vi "getSheetDim.vi"(8 "error in (no error)":errorcluster, 10 "Refnum Cluster Out":T1, 11 "reference in":refnum<class "excelFile.lvclass">) -> (0 "error out":errorcluster, 2 "rowNumber":i32, 3 "reference out":refnum<class "excelFile.lvclass">)   [LabVIEW 2015, in "excelFile.lvclass"]
uses:
  excelFile.lvclass
  <userlib>/Read_Excel_Values.llb/GetXL_CellValues_2D_String.vi
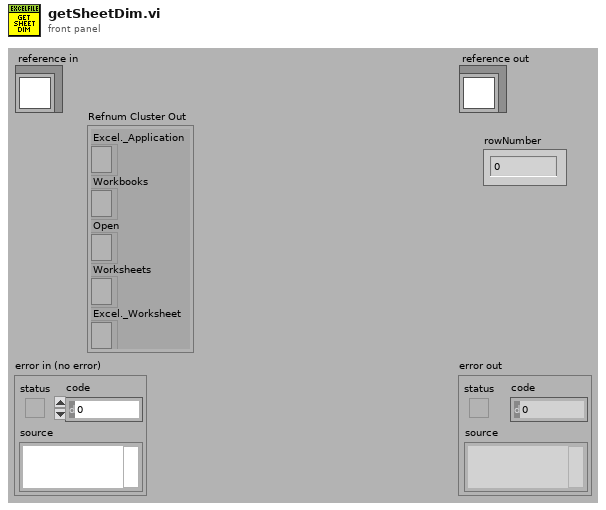
[diagram p1: front panel]
types:
  T1 = cluster{"Excel._Application":refnum<k7>, "Workbooks":refnum<k7>, "Open":refnum<k7>, "Worksheets":refnum<k7>, "Excel._Worksheet":refnum<k7>}
  T2 = typedef "excelFile.lvclass/ObjectAttributesRef.ctl" = refnum<data-value>
  T3 = typedef "excelFile.lvclass/ObjectAttributes.ctl" = cluster{"MyAttribute":dbl, "path":string, "Refnum Excel":cluster{"Excel._Application":refnum<k7>, "Workbooks":refnum<k7>, "Open":refnum<k7>}, "data":string[][][], "fileType":T4, "sheetName":string[]}
  T4 = typedef "excelFile.lvclass/fileType.ctl" = enum16{"database", "CosmedTest"}
  T5 = cluster{"Excel._Application":refnum<k7>, "Workbooks":refnum<k7>, "Open":refnum<k7>}
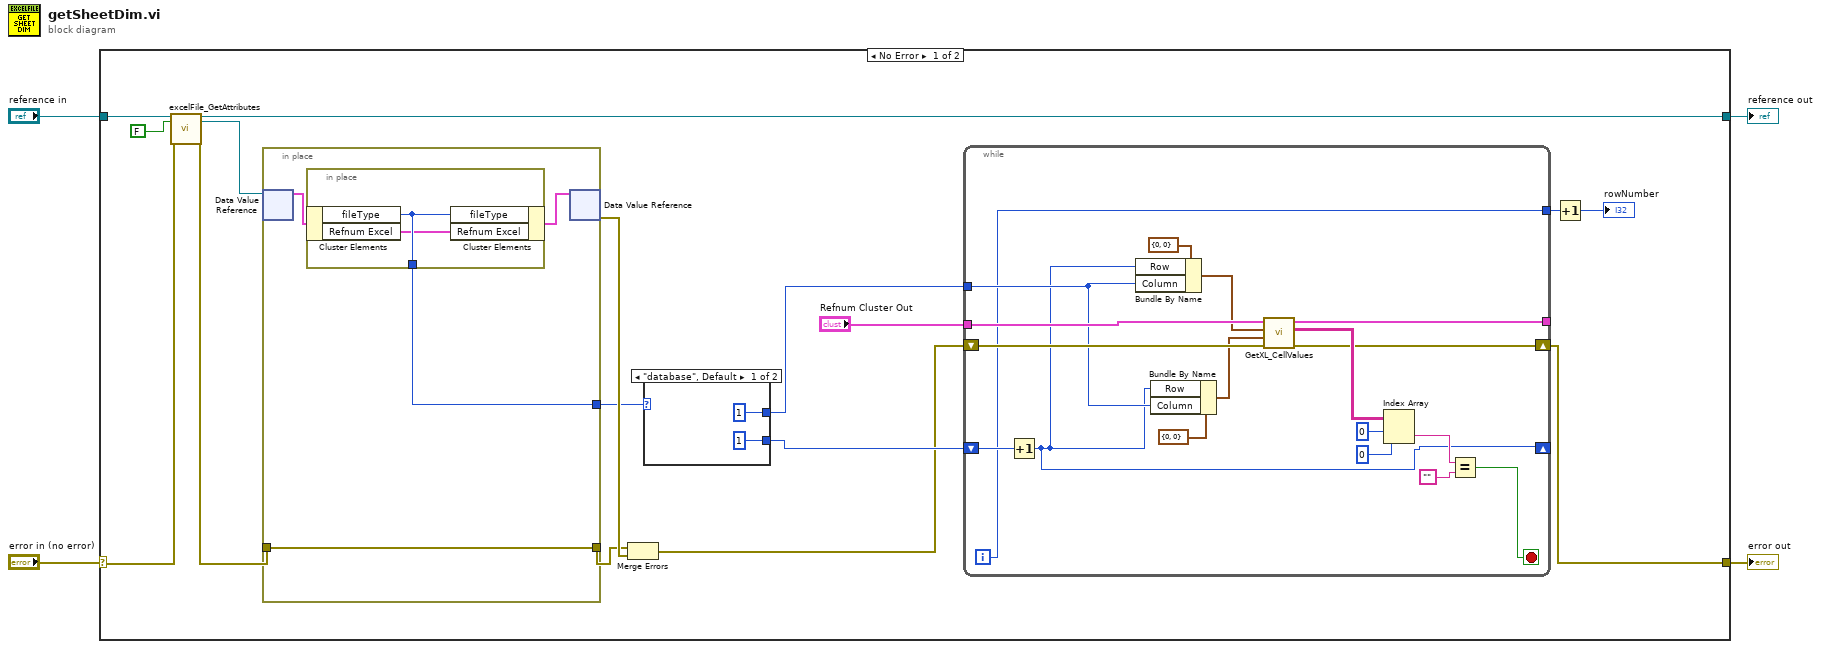
[diagram p0: block diagram]
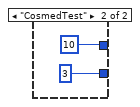
[diagram p2: hidden frame]
diagram:
  n1 = case shown="No Error" "error in (no error)" {
    selector: "error in (no error)" -> [w16 w50]
    tunnel: [w10 w50] -> w3
    tunnel: [w12 w49] -> w1
    tunnel: "reference in" -> [w18 w49]
    frame No Error {
      n2 = call "excelFile_GetAttributes.vi"("reference in"=w18, "return data? (T)"=FALSE, "error in (no error)"=w16) -> ("reference out"=w12:refnum<class "excelFile.lvclass">, "attributes ref"=w14:T2, "error out"=w15:errorcluster)  [unwired: 13 in, 1 out]
      n3 = in-place {
        in-place-border: w15 -> [w44]
        in-place-border: [w44] -> w19
        in-place-border: [w43] -> w11
        n4 = in-place-dvr #1(w14) -> (w45:T3)  [unwired: 1 out]
        n5 = in-place {
          in-place-border: [w48] -> w43
          n6 = in-place-cluster #2(w45) -> ("fileType"=w48:T4, "Refnum Excel"=w47:T5)
          n7 = in-place-cluster #2("fileType"=w48, "Refnum Excel"=w47) -> (w46:T3)
        }
        n8 = in-place-dvr #1(w46) -> (w20:errorcluster)  [unwired: 1 out]
      }
      n9 = Merge Errors(w19, w20) -> (w7:errorcluster)
      n10 = case shown="\"database\", Default" w11 {
        tunnel: [1 10] -> w9
        tunnel: [1 3] -> w8
        frame "database", Default {
        }
        frame "CosmedTest" {
        }
      }
      n11 = while {
        tunnel: [w31] -> _
        shift-right: [w29] -> w10
        shift-left: w7 -> [w34]
        tunnel: [w25] -> w6
        tunnel: "Refnum Cluster Out" -> [w35]
        tunnel: w9 -> [w28]
        shift-right: [w26] -> _
        shift-left: w8 -> [w27]
        i -> [w25]
        stop <- w36 stop-if-true
        n12 = Increment(x=w27) -> (x+1=w26:i32)
        n13 = Bundle By Name(cluster=cluster{"Column":i32, "Row":i32} {"Column"=0, "Row"=0} ("Start"), "Row"=w26, "Column"=w28) -> (w33:cluster{"Column":i32, "Row":i32})
        n14 = Bundle By Name(cluster=cluster{"Column":i32, "Row":i32} {"Column"=0, "Row"=0} ("End"), "Row"=w26, "Column"=w28) -> (w32:cluster{"Column":i32, "Row":i32})
        n15 = call-poly <userlib>:"GetXL_CellValues.vi"("error in"=w34, "End"=w32, "Start"=w33, "Refnum Cluster In"=w35) -> ("error out"=w29:errorcluster, "data"=w30:string[][], "Refnum Cluster Out"=w31:T1)  [unwired: 5 in]
        n16 = Index Array(array=w30, index (row)=0, index (col)=0 ("disabled index (col)")) -> (element=w37:string)
        n17 = Equal?(x=w37, y="") -> (x = y?=w36:bool)
      }
      n18 = Increment(x=w6) -> (x+1=→"rowNumber":i32)
    }
    frame Error {
    }
  }
  "error out" <- w3
  "reference out" <- w1
